vi "autocorrelation.vi"() -> ()   [LabVIEW 2012]
uses:
  <vilib>/Analysis/6fits.llb/Curve Fitting Criteria.ctl
  <vilib>/Analysis/NI_AALPro.lvlib
panel:
  out "Normal part R":dbl format="%#_3g"
  out "Normal part diff":dbl format="%#_3g"
  out "AP part":dbl format="%#_3g"
  out "Normal part Int":dbl format="%#_3f"
  out "Countrate":dbl format="%#_3p"
  out "amplitude":dbl format="%#_3p"
  out "Waveform Chart":cluster{dbl, dbl, dbl}(graph)
  in  "Histogram Start 1 (ns)":i32=16
  in  "number":i32(ring) items=["Channel3"=2, "Channel2"=1, "Channel1"=0]
  out "Single Count Channel3":dbl format="%#_3p"
  out "Single Count Channel2":dbl format="%#_3p"
  in  "i last":i32
  in  "Reset 1":bool
  in  "Histogram Bin":string(combo)="0"
  in  "Channel3 Pulse Front":string(combo)
  in  "Channel2 Pulse Front":string(combo)
  out "Waveform Graph 1":cluster{dbl, dbl, dbl[][]}(graph) caption="Waveform Graph"
  out "Single Count Channel1":dbl format="%#_3p"
  out "Exposition time (ms)":i64
  out "Measurement index":i64
  out "Start OK":bool
  in  "Exit":bool
  in  "Channel3 Threshold Voltage (mV)":i32
  in  "Channel2 Threshold Voltage (mV)":i32
  in  "Channel1 Pulse Front":string(combo)
  in  "Channel1 Threshold Voltage (mV)":i32 min=0 max=5000 step=10
  in  "Exposition Time (ms)":i64
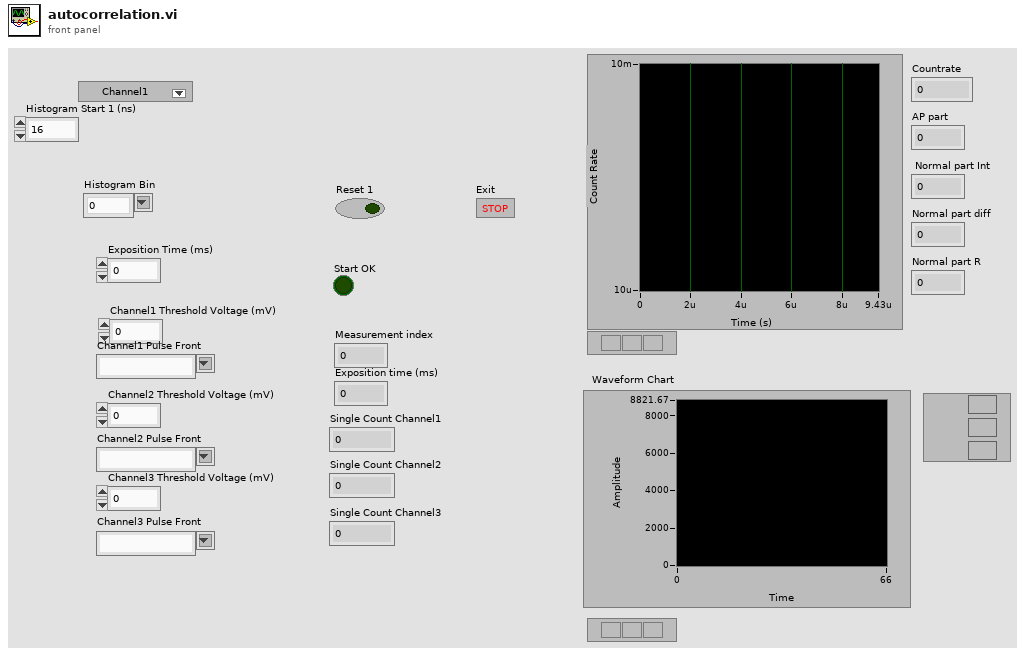
[diagram p1: front panel]
types:
  T1 = cluster{"Channel1":bool, "Channel2":bool, "Channel3":bool, "Channel4":bool}
  T2 = cluster{"[0]":i64, "Channel1 Threshold Voltage (mV)":i32, "Channel1 Pulse Front":string, "Channel2 Threshold Voltage (mV)":i32, "Channel2 Pulse Front":string, "Channel3 Threshold Voltage (mV)":i32, "Channel3 Pulse Front ":string, "Channel4 Threshold Voltage (mV)":i32, "Channel4 Pulse Front ":string, "Single Count Enable":cluster{"Channel1":bool, "Channel2":bool, "Channel3":bool, "Channel4":bool}, "Single Count Max":i32, "Sum Count Enable":cluster{"Channel1":bool, "Channel2":bool, "Channel3":bool, "Channel4":bool}, "Sum Count Max":i32, "Start-Stop1 Multyplex":cluster{"Stop Channel":string, "Start Channel":string}, "Stop Delay 1 (ns)":i16, "Window Length 1 (ns)":i32, "Window Offset 1 (ns) ":i32, "Conditional Correlation 1":string, "Histogram Bin 1":string, "Histogram Start 1 (ns) ":i32, "Start-Stop2 Multyplex ":cluster{"Stop Channel":string, "Start Channel":string}, "Stop Delay 2 (ns)":i16, "Window Length 2 (ns) ":i32, "Window Offset 2 (ns) ":i32, "Conditional Correlation 2":string, "Histogram Bin 2":string, "Histogram Start 2 (ns)  ":i32, "Start-Stop3 Multyplex":cluster{"Stop Channel":string, "Start Channel":string}, "Stop Delay 3 (ns)":i16, "Window Length 3 (ns) ":i32, "Window Offset 3 (ns) ":i32, "Conditional Correlation 3":string, "Histogram Bin 3":string, "Histogram Start 3 (ns) ":i32, "Start-Stop4 Multyplex":cluster{"Stop Channel":string, "Start Channel":string}, "Stop Delay 4 (ns)":i16, "Window Length 4 (ns)  ":i32, "Window Offset 4 (ns) ":i32, "Conditional Correlation 4":string, "Histogram Bin 4":string, "Histogram Start 4 (ns)  ":i32, "Coincidence Count Enable":cluster{"Start-Stop1":bool, "Start-Stop2":bool, "Start-Stop3":bool, "Start-Stop4":bool}, "Coincidence Count Max":i32, "Coincidence Sum Enable":cluster{"Start-Stop1":bool, "Start-Stop2":bool, "Start-Stop3":bool, "Start-Stop4":bool}, "Coincidence Sum Max":i32, "Output Channel Enable":cluster{"Channel1":bool, "Channel2":bool, "Channel3":bool, "Channel4":bool}, "Output Channel Inversion":cluster{"Channel1":bool, "Channel2":bool, "Channel3":bool, "Channel4":bool, "Output":bool}}
  T3 = typedef "NI_AALPro.lvlib/Curve Fitting Criteria.ctl" = u16
  T4 = cluster{"Going":bool, "Iinterrupted":bool, "Timer stop":bool, "Single count stop Ch1":bool, "Single count stop Ch2":bool, "Single count stop Ch3":bool, "Single count stop Ch4":bool, "Sum count stop":bool, "Coincidence count stop SS1":bool, "Coincidence count stop SS2":bool, "Coincidence count stop SS3":bool, "Coincidence count stop SS4":bool, "Coincidence sum count stop":bool, "Reserved":bool, "Correlator is not initialised":bool, "Internal error":bool}
  T5 = cluster{"Measurement index":i64, "Exposition time (ms)":i64, "Single Count Channel1":i64, "Single Count Channel2":i64, "Single Count Channel3":i64, "Single Count Channel4":i64, "Sum Single Count":i64, "Coincidence Count SS1":i64, "Coincidence Count SS2":i64, "Coincidence Count SS4":i64, "Coincidence Count SS5":i64, "Sum Coincidence Count":i64}
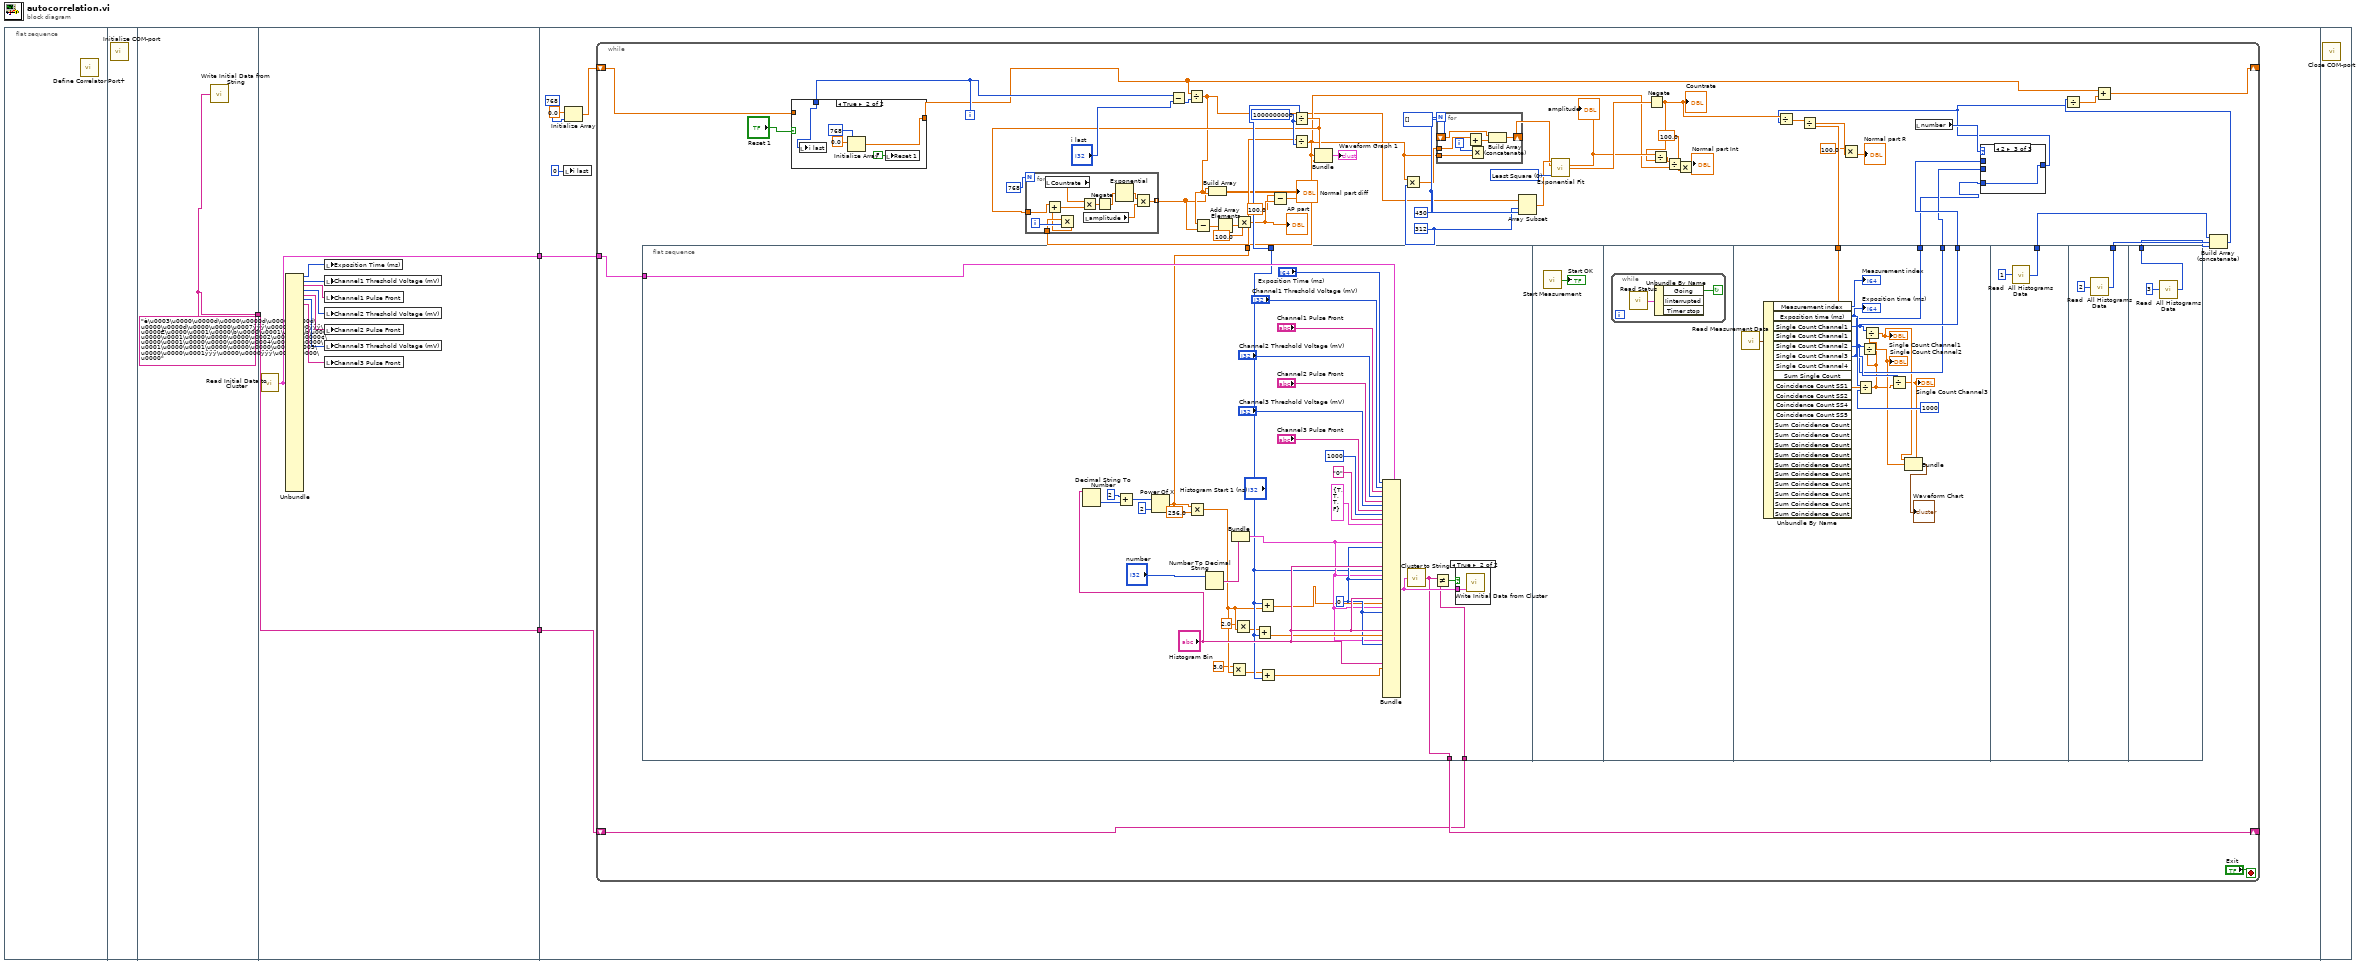
[diagram p0: block diagram]
diagram:
  n1 = flat-sequence {
    tunnel: [w4] -> w1
    tunnel: [w13] -> w3
    tunnel: [w5] -> w2
    tunnel: w1 -> [w5]
    tunnel: w3 -> [w19]
    tunnel: w2 -> [w15]
    frame #0 {
      n2 = call "Define Correlator Port+.vi"() -> ()  [unwired: 3 in]
    }
    frame #1 {
      n3 = call "Initialize COM-port.vi"() -> ()  [unwired: 4 in]
    }
    frame #2 {
      w4 = "è\u0003\u0000\u0000d\u0000\u0000d\u0000\u0000d\u0000\u0000d\u0000\u0000\u0007ÿÿÿ\u0000\u0000ÿÿÿ\u0000€\u0000\u0001\u0000\b\u0000\u0001\u0005\b\u0000‘\u0000\u0001\u0000\u0000\u0000\u0002\u0005\b\u0000¢\u0000\u0001\u0000\u0000\u0000\u0004\u0005\b\u0000\u0001\u0000\u0001\u0000\u0000\u0000\u0010\u0005\u0000\u0000\u0001ÿÿÿ\u0000\u0000ÿÿÿ\u0000\u0000\u0000" ("string")
      n4 = call "Write Initial Data from String.vi"("Data"=w4) -> ()  [unwired: 1 out]
    }
    frame #3 {
      n5 = call "Read Initial Data to Cluster.vi"() -> ("Correlator Initial Data 2"=w13:T2)  [unwired: 2 in]
      n6 = Unbundle(w13) -> ("[0]"=w12:i64, "Channel1 Threshold Voltage (mV)"=w11:i32, "Channel1 Pulse Front"=w10:string, "Channel2 Threshold Voltage (mV)"=w9:i32, "Channel2 Pulse Front"=w7:string, "Channel3 Threshold Voltage (mV)"=w8:i32, "Channel3 Pulse Front"=w6:string)  [unwired: 40 out]
      n7 = local write "Exposition Time (ms)"(w12) -> ()
      n8 = local write "Channel1 Threshold Voltage (mV)"(w11) -> ()
      n9 = local write "Channel1 Pulse Front"(w10) -> ()
      n10 = local write "Channel2 Threshold Voltage (mV)"(w9) -> ()
      n11 = local write "Channel2 Pulse Front"(w7) -> ()
      n12 = local write "Channel3 Threshold Voltage (mV)"(w8) -> ()
      n13 = local write "Channel3 Pulse Front"(w6) -> ()
    }
    frame #4 {
      n14 = local write "i last"(0 ("i last")) -> ()
      n15 = Initialize Array(0.0 ("element"), 768 ("dimension size")) -> (w16:dbl[])
      n16 = while {
        tunnel: w19 -> [w74]
        shift-right: [w68] -> _
        shift-left: w16 -> [w66]
        shift-right: [w72] -> _
        shift-left: w15 -> [w71]
        i -> [w64]
        stop <- "Exit" stop-if-true
        w52 = T3 0 items=["Least Square", "Least Absolute Residual", "Bisquare"] ("method")
        w49 = 450 ("length")
        w48 = 312 ("index")
        w69 = 1000000000 ("y")
        n17 = flat-sequence {
          tunnel: w74 -> [w132]
          tunnel: ["Histogram Start 1 (ns)"] -> w70
          tunnel: [w123] -> w72
          tunnel: w71 -> [w125]
          tunnel: [w114] -> w50
          tunnel: [w147] -> w55
          tunnel: [w149] -> w54
          tunnel: [w148] -> w56
          tunnel: [w142] -> w23
          tunnel: [w154] -> w61
          tunnel: [w156] -> w59
          tunnel: [w158] -> w58
          frame #0 {
            w112 = i16 0 ("Stop Delay1  (ns)")
            n18 = Decimal String To Number(string="Histogram Bin") -> (number=w120:i32)  [unwired: 2 in, 1 out]
            n19 = Add(x=2, y=w120) -> (x+y=w119:i32)
            n20 = Power Of X(1:i8 2 ("x"), 2:w119) -> (0:w114:dbl)
            n21 = Multiply(x=w114, y=256.0) -> (x*y=w108:dbl)
            n22 = Number To Decimal String(number="number") -> (decimal integer string=w121:string)  [unwired: 1 in]
            n23 = Multiply(x=3.0, y=w108) -> (x*y=w105:dbl)
            n24 = Bundle(w121, w121) -> (w111:cluster{string, string})  [unwired: 1 in]
            n25 = Multiply(x=2.0, y=w108) -> (x*y=w107:dbl)
            n26 = Add(x=w107, y="Histogram Start 1 (ns)") -> (x+y=w115:dbl)
            n27 = Add(x="Histogram Start 1 (ns)", y=w108) -> (x+y=w103:dbl)
            n28 = Add(x=w105, y="Histogram Start 1 (ns)") -> (x+y=w109:dbl)
            n29 = Bundle(cluster=w132, "[0]"="Exposition Time (ms)", "Channel1 Threshold Voltage (mV)"="Channel1 Threshold Voltage (mV)", "Channel1 Pulse Front"="Channel1 Pulse Front", "Channel2 Threshold Voltage (mV)"="Channel2 Threshold Voltage (mV)", "Channel2 Pulse Front"="Channel2 Pulse Front", "Channel3 Threshold Voltage (mV)"="Channel3 Threshold Voltage (mV)", "Channel3 Pulse Front"="Channel3 Pulse Front", "Channel4 Threshold Voltage (mV)"=1000, "Channel4 Pulse Front"="0", "Single Count Enable"=T1 {"Channel1"=TRUE, "Channel2"=TRUE, "Channel3"=TRUE, "Channel4"=FALSE}, "Start-Stop1 Multyplex"=w111, "Stop Delay 1 (ns)"=w112, "Histogram Bin 1"="Histogram Bin", "Histogram Start 1 (ns)"="Histogram Start 1 (ns)", "Start-Stop2 Multyplex"=w111, "Stop Delay 2 (ns)"=w112, "Histogram Bin 2"="Histogram Bin", "Histogram Start 2 (ns)"=w103, "Start-Stop3 Multyplex"=w111, "Stop Delay 3 (ns)"=w112, "Histogram Bin 3"="Histogram Bin", "Histogram Start 3 (ns)"=w115, "Start-Stop4 Multyplex"=w111, "Stop Delay 4 (ns)"=w112, "Histogram Bin 4"="Histogram Bin", "Histogram Start 4 (ns)"=w109) -> (w126:T2)  [unwired: 21 in]
            n30 = call "Cluster to String.vi"("Correlator Initial Data"=w126) -> ("string"=w123:string)
            n31 = Not Equal?(x=w123, y=w125) -> (x != y?=w124:bool)
            n32 = case shown="True" w124 {
              tunnel: w126 -> [_ w138]
              frame False {
              }
              frame True {
                n33 = call "Write Initial Data from Cluster.vi"("Correlator Initial Data"=w138) -> ()  [unwired: 2 in, 1 out]
              }
            }
          }
          frame #1 {
            n34 = call "Start Measurement.vi"() -> ("Start OK"=→"Start OK":bool)  [unwired: 2 in]
          }
          frame #2 {
            n35 = while {
              stop <- w140 continue-if-true
              n36 = call "Read Status.vi"() -> ("Status Data"=w141:T4)  [unwired: 2 in]
              n37 = Unbundle By Name(w141) -> ("Going"=w140:bool)  [unwired: 2 out]
            }
          }
          frame #3 {
            n38 = call "Read Measurement Data.vi"() -> ("Measurement Data"=w152:T5)  [unwired: 3 in]
            n39 = Unbundle By Name(w152) -> ("Measurement index"=→"Measurement index":i64, "Exposition time (ms)"=w151:i64, "Single Count Channel1"=w148:i64, "Single Count Channel2"=w147:i64, "Single Count Channel3"=w149:i64)  [unwired: 17 out]
            "Exposition time (ms)" <- w151
            n40 = Divide(x=w151, y=1000) -> (x/y=w142:dbl)
            n41 = Divide(x=w147, y=w142) -> (x/y=w145:dbl)
            "Single Count Channel2" <- w145
            n42 = Divide(x=w148, y=w142) -> (x/y=w146:dbl)
            "Single Count Channel1" <- w146
            n43 = Divide(x=w149, y=w142) -> (x/y=w144:dbl)
            "Single Count Channel3" <- w144
            n44 = Bundle(w146, w145, w144) -> (→"Waveform Chart":cluster{dbl, dbl, dbl})  [unwired: 1 in]
          }
          frame #4 {
            n45 = call "Read  All Histograms Data.vi"("Start-Stop#"=i8 1) -> ("Array"=w154:i64[])
          }
          frame #5 {
            n46 = call "Read  All Histograms Data.vi"("Start-Stop#"=i8 2) -> ("Array"=w156:i64[])
          }
          frame #6 {
            n47 = call "Read  All Histograms Data.vi"("Start-Stop#"=i8 3) -> ("Array"=w158:i64[])
          }
        }
        n48 = case shown="True" "Reset 1" {
          tunnel: w66 -> [w97 _]
          tunnel: [w97 w98] -> w53
          tunnel: w64 -> [_ w99]
          frame False {
          }
          frame True {
            n49 = local write "i last"(w99) -> ()
            n50 = Initialize Array(0.0 ("element"), 768 ("dimension size")) -> (w98:dbl[])
            n51 = local write "Reset 1"(FALSE ("Reset")) -> ()
          }
        }
        n52 = Subtract(x=w64, y="i last") -> (x-y=w62:i32)
        n53 = Divide(x=w53, y=w62) -> (x/y=w34:dbl[])
        n54 = Divide(x=w70, y=w69) -> (x/y=w37:dbl)
        n55 = Divide(x=w50, y=w69) -> (x/y=w36:dbl)
        n56 = for {
          N: 768 -> [_]
          tunnel: w37 -> [w86]
          tunnel: w36 -> [w84]
          tunnel: [w77] -> w33 mode=indexing
          i -> [w85]
          n57 = local read "Countrate"() -> (w81:dbl)
          n58 = Multiply(x=w84, y=w85) -> (x*y=w83:dbl)
          n59 = Add(x=w86, y=w83) -> (x+y=w82:dbl)
          n60 = Multiply(x=w81, y=w82) -> (x*y=w80:dbl)
          n61 = local read "amplitude"() -> (w78:dbl)
          n62 = Negate(x=w80) -> (-x=w76:dbl)
          n63 = Exponential(1:w76) -> (0:w79:dbl)
          n64 = Multiply(x=w79, y=w78) -> (x*y=w77:dbl)
        }
        n65 = Subtract(x=w34, y=w33) -> (x-y=w32:dbl[])
        n66 = Build Array(w33, w34) -> (w35:dbl[][])
        n67 = Add Array Elements(numeric array=w32) -> (sum=w31:dbl)
        n68 = Multiply(x=100.0, y=w31) -> (x*y=w29:dbl)
        "AP part" <- w29
        n69 = Subtract(x=100.0, y=w29) -> (x-y=→"Normal part diff":dbl)
        n70 = Bundle(w37, w36, w35) -> (→"Waveform Graph 1":cluster{dbl, dbl, dbl[][]})  [unwired: 1 in]
        n71 = Multiply(x=w36, y=w48) -> (x*y=w47:dbl)
        n72 = for {
          N: w49 -> [_]
          tunnel: w47 -> [w89]
          shift-right: [w92] -> w39
          shift-left: i32[] [] -> [w90]
          tunnel: w36 -> [w87]
          i -> [w93]
          n73 = Multiply(x=w93, y=w87) -> (x*y=w88:dbl)
          n74 = Add(x=w89, y=w88) -> (x+y=w91:dbl)
          n75 = Build Array (concatenate)(w90, w91) -> (w92:dbl[])
        }
        n76 = Array Subset(array=w34, index=w48, length=w49) -> (w40:dbl[])
        n77 = call <vilib>:"Exponential Fit.vi"("Y"=w40, "X"=w39, "method"=w52) -> ("amplitude"=w43:dbl, "damping"=w46:dbl)  [unwired: 7 in, 4 out]
        "amplitude" <- w43
        n78 = Negate(x=w46) -> (-x=w26:dbl)
        "Countrate" <- w26
        n79 = Divide(x=w43, y=w26) -> (x/y=w45:dbl)
        n80 = Divide(x=w45, y=w36) -> (x/y=w44:dbl)
        n81 = Multiply(x=w44, y=100.0) -> (x*y=→"Normal part Int":dbl)
        n82 = local read "number"() -> (w57:i32)
        n83 = case shown="2" w57 {
          tunnel: [w94 w95 w96] -> w25
          tunnel: w56 -> [w94 _ _]
          tunnel: w55 -> [_ w95 _]
          tunnel: w54 -> [_ _ w96]
          frame 0, Default {
          }
          frame 1 {
          }
          frame 2 {
          }
        }
        n84 = Divide(x=w26, y=w25) -> (x/y=w24:dbl)
        n85 = Divide(x=w24, y=w23) -> (x/y=w22:dbl)
        n86 = Multiply(x=100.0, y=w22) -> (x*y=→"Normal part R":dbl)
        n87 = Build Array (concatenate)(w61, w59, w58) -> (w60:i64[])
        n88 = Divide(x=w60, y=w25) -> (x/y=w67:dbl[])
        n89 = Add(x=w53, y=w67) -> (x+y=w68:dbl[])
      }
    }
    frame #5 {
      n90 = call "Close COM-port.vi"() -> ()  [unwired: 4 in]
    }
  }
